vi "Last Year Is Leap Year.vi"() -> (3 "Last Year Is Leap Year":bool)   [LabVIEW 2024]
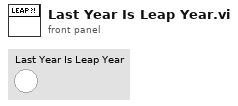
[diagram p1: front panel]
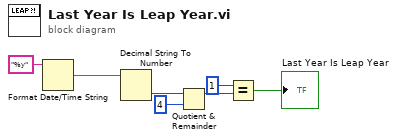
[diagram p0: block diagram]
diagram:
  n1 = Format Date/Time String(time format string (%c)="%y") -> (date/time string=w6:string)  [unwired: 2 in]
  n2 = Decimal String To Number(string=w6) -> (number=w5:i32)  [unwired: 2 in, 1 out]
  n3 = Quotient & Remainder(x=w5, y=4) -> (x-y*floor(x/y)=w3:i32)  [unwired: 1 out]
  n4 = Equal?(x=1, y=w3) -> (x = y?=→"Last Year Is Leap Year":bool)
